vi "Set Up Dialog - Goniometer .vi"() -> ()   [LabVIEW 2012]
panel:
  in  "Done":bool
  # "iWorx - Goniometer - Set Up"
  # "Set Up Instructions"
  # "1. Connect the IX-MYDAQ adaptor board to the NI myDAQ.\n\n2. Connect the NI myDAQ to your computer using a USB cable.\n\n3. Connect the GNN-100 Goniometer to the IX-MYDAQ.\n\n4. Use a text book to set the GNN-100 to an angle of 90°, type 90 for the SP1 Angle and press set to record the voltage in SP1 Voltage.\n\n5. Set the GNN-100 straight, enter '0' for SP2 Angle, then press Set to record the voltage in SP2 Voltage."
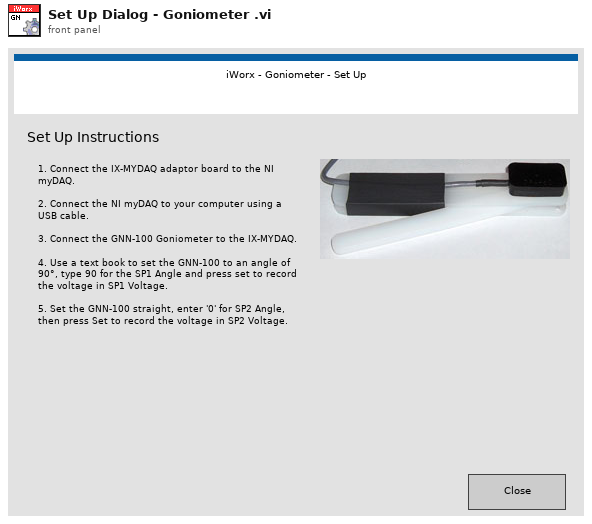
[diagram p1: front panel]
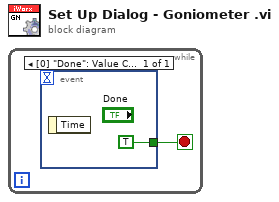
[diagram p0: block diagram]
diagram:
  n1 = while {
    stop <- w1 stop-if-true
    n2 = event shown="[0] \"Done\": Value Change;  Panel Close" {
      selector: _ -> [_]
      dyn-events: _ -> [_]
      timeout: _ -> [_]
      tunnel: [TRUE] -> w1
      event "Done": Value Change; Panel Close {
        n3 = event-data() -> ()  [unwired: 1 in, 1 out]
      }
    }
  }
